vi "Process Image for Target.vi"(0 "Src Image":T2, 1 "Color Mode":u16(ring)=2 items=["RGB", "HSL", "HSV", "HSI"], 9 "Color Components":T3={"Hue"={110.0, 142.0}, "Sat"={138.0, 255.0}, "Val"={139.0, 198.0}} {"Val" scale=0.0..255.0; "Sat" scale=0.0..255.0; "Hue" scale=0.0..255.0 scale format="%#_3g"}, 11 "Area Cutoff %":dbl=0.05) -> (4 "Src Image Out":T2, 8 "Threshold":T2, 15 "Particles":T1(array[cluster]))   [LabVIEW 2013]
doc: "Use color, rectangularity, and aspect ratio to identify and describe potential strips of retroreflective material within the image."
uses:
  <vilib>/vision/Image Controls.llb/IMAQ Image.ctl
  <vilib>/vision/NI_Vision_Development_Module.lvlib
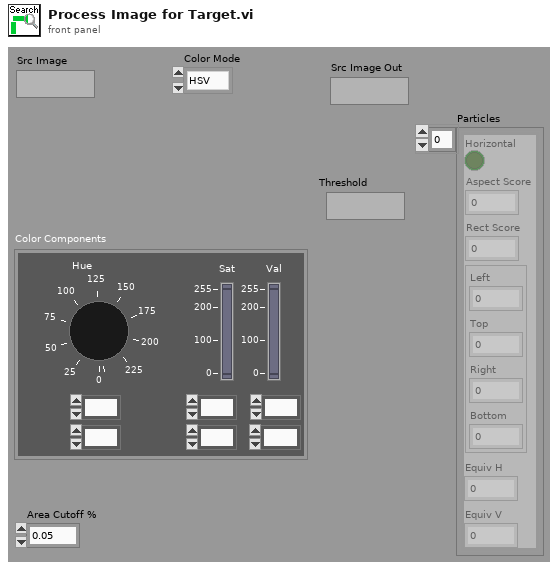
[diagram p1: front panel]
types:
  T1 = cluster{"Horizontal":bool, "Aspect Score":dbl, "Rect Score":dbl, cluster{"Left":dbl, "Top":dbl, "Right":dbl, "Bottom":dbl}, "Equiv H":dbl, "Equiv V":dbl}[]
  T2 = typedef "IMAQ Image.ctl" = refnum<image>
  T3 = cluster{"Hue":cluster{dbl, dbl}, "Sat":cluster{dbl, dbl}, "Val":cluster{dbl, dbl}}
  T4 = typedef "Particle Parameters" = i32
  T5 = typedef "Image Type" = u32
  T6 = cluster{"Horizontal":bool, "Score":dbl, "Score":dbl, cluster{"Numeric":dbl, "Numeric":dbl, "Numeric":dbl, "Numeric":dbl}, "Numeric":dbl, "Numeric":dbl}[]
  T7 = cluster{"Numeric":dbl, "Numeric":dbl, "Numeric":dbl, "Numeric":dbl}
  T8 = cluster{"Horizontal":bool, "Score":dbl, "Score":dbl, cluster{"Numeric":dbl, "Numeric":dbl, "Numeric":dbl, "Numeric":dbl}, "Numeric":dbl, "Numeric":dbl}
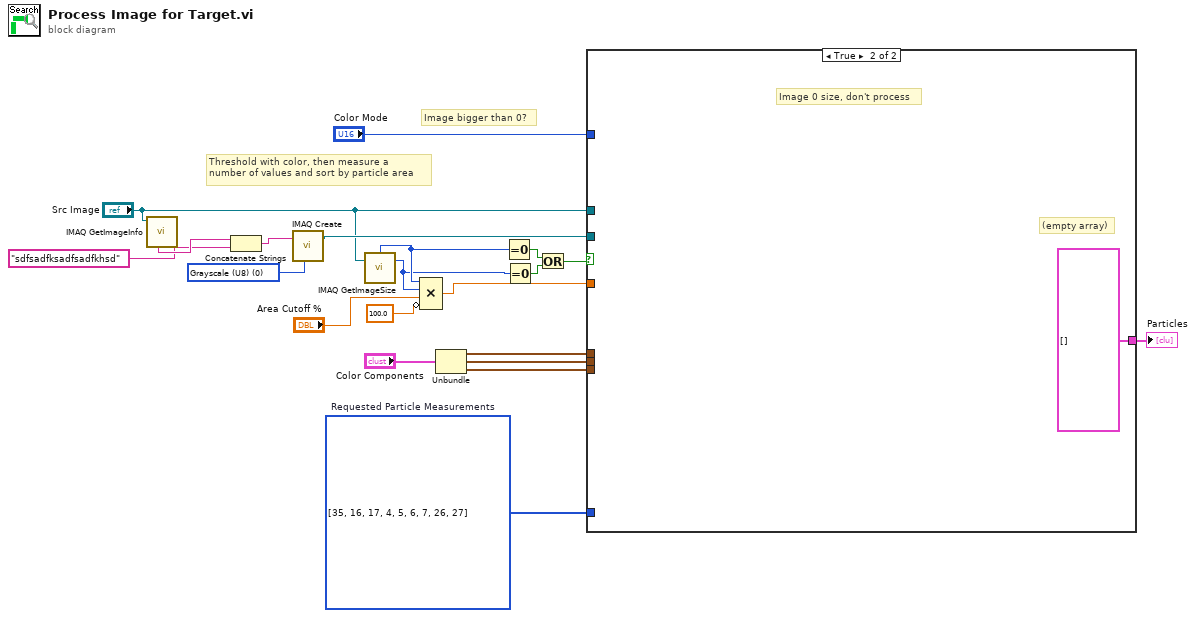
[diagram p0: block diagram]
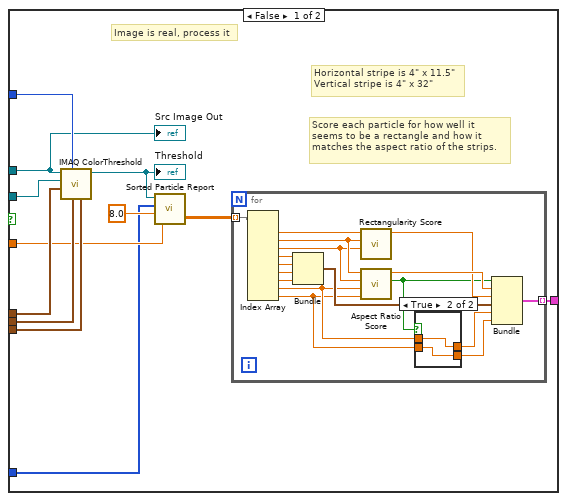
[diagram p2: hidden frame]
diagram:
  w11 = T4[] [35, 16, 17, 4, 5, 6, 7, 26, 27] items=["Center of Mass X", "Center of Mass Y", "First Pixel X", "First Pixel Y", "Bounding Rect Left", "Bounding Rect Top", "Bounding Rect Right", "Bounding Rect Bottom", "Max Feret Diameter Start X", "Max Feret Diameter Start Y", "Max Feret Diameter End X", "Max Feret Diameter End Y", "Max Horiz. Segment Length Left", "Max Horiz. Segment Length Right", "Max Horiz. Segment Length Row", "-", "Bounding Rect Width", "Bounding Rect Height", "Bounding Rect Diagonal", "Perimeter", "Convex Hull Perimeter", "Holes' Perimeter", "Max Feret Diameter", "Equivalent Ellipse Major Axis", "Equivalent Ellipse Minor Axis", "Equivalent Ellipse Minor Axis (Feret)", "Equivalent Rect Long Side", "Equivalent Rect Short Side", "Equivalent Rect Diagonal", "Equivalent Rect Short Side (Feret)", "Average Horiz. Segment Length", "Average Vert. Segment Length", "Hydraulic Radius", "Waddel Disk Diameter", "-", "Area", "Holes' Area", "Particle & Holes' Area", "Convex Hull Area", "Image Area", "-", "Number of Holes", "Number of Horiz. Segments", "Number of Vert. Segments", "-", "Orientation", "Max Feret Diameter Orientation", "-", "% Area/Image Area", "% Area/(Particle & Holes' Area)", "Ratio of Equivalent Ellipse Axes", "Ratio of Equivalent Rect Sides", "-", "Elongation Factor", "Compactness Factor", "Heywood Circularity Factor", "Type Factor", "-", "Sum X", "Sum Y", "Sum XX", "Sum XY", "Sum YY", "Sum XXX", "Sum XXY", "Sum XYY", "Sum YYY", "-", "Moment of Inertia XX", "Moment of Inertia XY", "Moment of Inertia YY", "Moment of Inertia XXX", "Moment of Inertia XXY", "Moment of Inertia XYY", "Moment of Inertia YYY", "Norm. Moment of Inertia XX", "Norm. Moment of Inertia XY", "Norm. Moment of Inertia YY", "Norm. Moment of Inertia XXX", "Norm. Moment of Inertia XXY", "Norm. Moment of Inertia XYY", "Norm. Moment of Inertia YYY", "Hu Moment 1", "Hu Moment 2", "Hu Moment 3", "Hu Moment 4", "Hu Moment 5", "Hu Moment 6", "Hu Moment 7"]  # Requested Particle Measurements
  w17 = T5 0 items=["Grayscale (U8)", "Grayscale (I16)", "Grayscale (SGL)", "Complex (CSG)", "RGB (U32)", "HSL (U32)", "RGB (U64)", "Grayscale (U16)"] ("Image Type")
  # "Image bigger than 0?"
  # "Threshold with color, then measure a\nnumber of values and sort by particle area"
  n1 = call "IMAQ GetImageInfo"("Image"="Src Image") -> ("Image Name"=w8:string)  [unwired: 3 in, 7 out]
  n2 = Concatenate Strings(w8, "sdfsadfksadfsadfkhsd" ("string")) -> (w6:string)
  n3 = call "IMAQ Create"("Image Name"=w6, "Image Type"=w17) -> ("New Image"=w16:T2)  [unwired: 3 in, 1 out]
  n4 = call "IMAQ GetImageSize"("Image"="Src Image") -> ("Y Resolution"=w4:i32, "X Resolution"=w5:i32)  [unwired: 3 in, 1 out]
  n5 = Compound Arithmetic op=MULTIPLY(w5, w4, "Area Cutoff %", invert 100.0 ("value")) -> (w13:dbl)
  n6 = Unbundle("Color Components") -> ("Hue"=w18:cluster{dbl, dbl}, "Sat"=w19:cluster{dbl, dbl}, "Val"=w20:cluster{dbl, dbl})
  n7 = Equal To 0?(x=w5) -> (x = 0?=w3:bool)
  n8 = Equal To 0?(x=w4) -> (x = 0?=w2:bool)
  n9 = Or(x=w3, y=w2) -> (x .or. y?=w1:bool)
  n10 = case shown="True" w1 {
    tunnel: w20 -> [w33 _]
    tunnel: w19 -> [w32 _]
    tunnel: w18 -> [w31 _]
    tunnel: w16 -> [w29 _]
    tunnel: w13 -> [w28 _]
    tunnel: "Color Mode" -> [w27 _]
    tunnel: w11 -> [w26 _]
    tunnel: [w23 T6 []] -> w10
    tunnel: "Src Image" -> [w22 _]
    frame False {
      # "Image is real, process it"
      # "Score each particle for how well it\nseems to be a rectangle and how it\nmatches the aspect ratio of the strips."
      # "Horizontal stripe is 4\" x 11.5\"\nVertical stripe is 4\" x 32\""
      n11 = call "IMAQ ColorThreshold"("Blue or Luma or Val or Inten Range"=w33, "Green or Sat Range"=w32, "Color Mode"=w27, "Red or Hue Range"=w31, "Image Dst"=w29, "Image Src"=w22) -> ("Image Dst Out"=w24:T2)  [unwired: 4 in, 1 out]
      "Threshold" <- w24
      n12 = call "Sorted Particle Report.vi"("Area Size Limit"=w28, "Particle Count Limit"=8.0, "Pixel Measurements"=w26, "Image in"=w24) -> ("Sorted Data"=w25:dbl[][])  [unwired: 1 out]
      n13 = for {
        tunnel: w25 -> [w50] mode=indexing
        tunnel: [w40] -> w23 mode=indexing
        n14 = Index Array(array=w50) -> (element #1=w49:dbl, element #2=w44:dbl, element #3=w43:dbl, element #4=w48:dbl, element #5=w47:dbl, element #6=w46:dbl, element #7=w45:dbl, element #8=w35:dbl, element #9=w34:dbl)  [unwired: 9 in]
        n15 = Bundle("Numeric"=w48, "Numeric"=w47, "Numeric"=w46, "Numeric"=w45) -> (w39:T7)  [unwired: 1 out]
        n16 = call "Rectangularity Score.vi"("Height"=w43, "Width"=w44, "Area"=w49) -> ("Score"=w41:dbl)  [unwired: 8 in]
        n17 = call "Aspect Ratio Score.vi"("Equivalent Rect Short"=w34, "Equivalent Rect Long"=w35, "Height"=w43, "Width"=w44) -> ("Horizontal"=w36:bool, "Score"=w42:dbl)  [unwired: 6 in]
        n18 = case shown="True" w36 {
          tunnel: w34 -> [w51 w54]
          tunnel: w35 -> [w52 w53]
          tunnel: [w52 w54] -> w38
          tunnel: [w51 w53] -> w37
          frame False {
          }
          frame True {
          }
        }
        n19 = Bundle("Horizontal"=w36, "Score"=w42, "Score"=w41, w39, "Numeric"=w37, "Numeric"=w38) -> (w40:T8)  [unwired: 1 out]
      }
      "Src Image Out" <- w22
    }
    frame True {
      # "(empty array)"
      # "Image 0 size, don't process"
    }
  }
  "Particles" <- w10
